vi "Read Non-Sequential Address.vi"(7 "Target IC (1-8)":u8, 8 "error in (no error)":errorcluster, 10 "Address":u16 format="%04x", 11 "FPGA Sim in":refnum<class "FPGA Sim.lvclass">) -> (0 "error out":errorcluster, 2 "Data":u16 format="%04x")   [LabVIEW 2020, in "Unit Tests.lvlib" / "FPGA Sim.lvclass"]
uses:
  FPGA Sim.lvclass
  FPGA Sim.lvclass/FPGA Sim.ctl
  Dependencies/Virtual Memory Unit/Virtual Memory Unit.lvclass
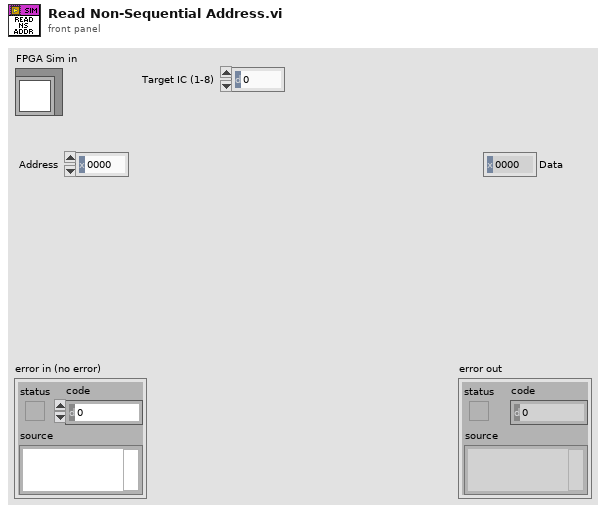
[diagram p1: front panel]
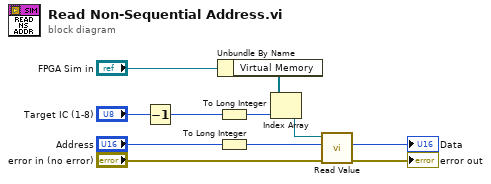
[diagram p0: block diagram]
diagram:
  n1 = Decrement(x="Target IC (1-8)") -> (x-1=w2:u8)
  n2 = Unbundle By Name("FPGA Sim in") -> ("Virtual Memory"=w9:refnum<class "Virtual Memory Unit.lvclass">[])
  n3 = To Long Integer(number=w2) -> (32bit integer=w8:i32)
  n4 = To Long Integer(number="Address") -> (32bit integer=w5:i32)
  n5 = Index Array(array=w9, index=w8) -> (element=w7:refnum<class "Virtual Memory Unit.lvclass">)
  n6 = call "Read Value.vi"("error in (no error)"="error in (no error)", "Index"=w5, "Virtual Memory Unit in"=w7) -> ("error out"=→"error out":errorcluster, "Value"=→"Data":u16)  [unwired: 7 in]
